vi "StringLogger.vi"(6 "Path Data":path, 8 "Error In":errorcluster, 9 "Function":string, 10 "Label":string, 11 "String to log":string) -> (0 "error out":errorcluster caption="Fehler (Ausgang)")   [LabVIEW 2020, in "hse-misc.lvlib"]
doc: "Simple helper VI for writing data to a log file. <b>Path Data</b> and <b>Label</b> form the folder structure, and <b>Function</b> is part of the file name.\n\n\n\n____\nHAMPEL SOFTWARE ENGINEERING v3.8.0 (2023-12-18 14:41)"
uses:
  hse-misc.lvlib
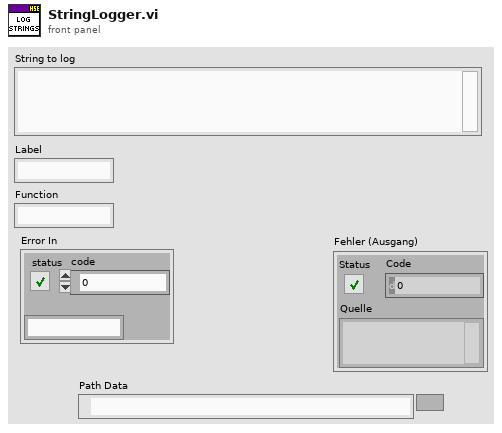
[diagram p1: front panel]
types:
  T1 = enum16{"open", "replace", "create", "open or create", "replace or create", "replace or create with confirmation"}
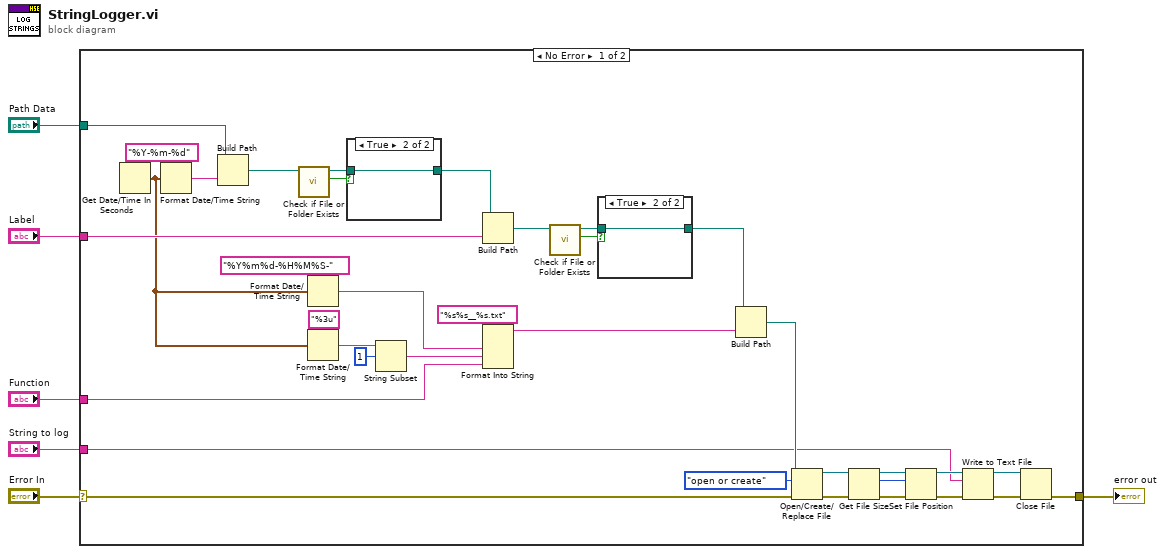
[diagram p0: block diagram]
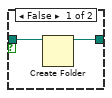
[diagram p2: hidden frame]
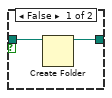
[diagram p3: hidden frame]
diagram:
  n1 = case shown="No Error" "Error In" {
    selector: "Error In" -> [w20 w49]
    tunnel: "Path Data" -> [w42 _]
    tunnel: "Label" -> [w39 _]
    tunnel: "String to log" -> [w9 _]
    tunnel: [w14 w49] -> w2
    tunnel: "Function" -> [w22 _]
    frame No Error {
      n2 = Get Date/Time In Seconds() -> (seconds since 1Jan1904=w29:timestamp)
      n3 = Format Date/Time String(time format string (%c)="%Y-%m-%d" ("Zeitformatierungs-String (%c)"), seconds (now)=w29) -> (date/time string=w40:string)  [unwired: 1 in]
      n4 = Build Path(base path=w42, name or relative path=w40) -> (appended path=w37:path)
      n5 = call <vilib>:"Check if File or Folder Exists.vi"("path"=w37) -> ("file or folder exists?"=w35:bool, "dup path"=w36:path)  [unwired: 8 in, 1 out]
      n6 = Format Date/Time String(time format string (%c)="%Y%m%d-%H%M%S-" ("Zeitformatierungs-String (%c)"), seconds (now)=w29) -> (date/time string=w27:string)  [unwired: 1 in]
      n7 = Format Date/Time String(time format string (%c)="%3u" ("Zeitformatierungs-String (%c)"), seconds (now)=w29) -> (date/time string=w25:string)  [unwired: 1 in]
      n8 = case shown="True" w35 {
        tunnel: w36 -> [w47 w48]
        tunnel: [w46 w48] -> w34
        frame False {
          n9 = Create Folder(path (use dialog)=w47) -> (created path=w46:path)  [unwired: 2 in, 2 out]
        }
        frame True {
        }
      }
      n10 = String Subset(string=w25, offset (0)=1 ("Offset (0)")) -> (substring=w24:string)  [unwired: 1 in]
      n11 = Build Path(base path=w34, name or relative path=w39) -> (appended path=w31:path)
      n12 = Format Into String(format string="%s%s__%s.txt" ("Format-String"), w27, w24, w22) -> (resulting string=w21:string)  [unwired: 2 in, 1 out]
      n13 = call <vilib>:"Check if File or Folder Exists.vi"("path"=w31) -> ("file or folder exists?"=w33:bool, "dup path"=w32:path)  [unwired: 8 in, 1 out]
      n14 = case shown="True" w33 {
        tunnel: w32 -> [w44 w45]
        tunnel: [w43 w45] -> w30
        frame False {
          n15 = Create Folder(path (use dialog)=w44) -> (created path=w43:path)  [unwired: 2 in, 2 out]
        }
        frame True {
        }
      }
      n16 = Build Path(base path=w30, name or relative path=w21) -> (appended path=w19:path)
      n17 = Open/Create/Replace File(file path (use dialog)=w19, error in=w20, operation (0:open)=T1."open or create") -> (refnum out=w13:refnum<file>, error out=w18:errorcluster)  [unwired: 3 in, 1 out]
      n18 = Get File Size(file=w13, error in=w18) -> (refnum out=w12:refnum<file>, size (in bytes)=w8:i64, 0:w17:errorcluster)
      n19 = Set File Position(offset (in bytes) (0)=w8, refnum=w12, error in=w17) -> (refnum out=w11:refnum<file>, error out=w16:errorcluster)  [unwired: 1 in]
      n20 = Write to Text File(file (use dialog)=w11, text=w9, error in=w16) -> (refnum out=w10:refnum<file>, error out=w15:errorcluster)  [unwired: 1 in, 1 out]
      n21 = Close File(refnum=w10, error in=w15) -> (error out=w14:errorcluster)  [unwired: 1 out]
    }
    frame Error {
    }
  }
  "error out" <- w2
